vi "Gui_SetupExperiment.vi"(7 "Variant for Path":variant, 8 "error in (no error)":errorcluster, 11 "Variant":variant) -> (0 "error out":errorcluster caption="sortie d'erreur", 3 "Variant Output":variant)   [LabVIEW 2017]
uses:
  controls/LASER_Inputs.ctl
  controls/EXPERIMENT_Inputs.ctl
  controls/EXPERT_Path_Selector.ctl
panel:
  in  "EXPERIMENT Inputs":T1={"Setup"="", "Date"="", "User Name"="", "Comment"="", "Experiment Procedures"=[], "Chemical Source"="", "Sample Components"=[], "Species"=[], "Laser 1"={"Used"=FALSE, "Name"="", "Reference"="", "Wavelength"=0.0, "Energy"=0.0}, "Laser 2"={"Used"=FALSE, "Name"="", "Reference"="", "Wavelength"=0.0, "Energy"=0.0}, "Laser 3"={"Used"=FALSE, "Name"="", "Reference"="", "Wavelength"=0.0, "Energy"=0.0}, "Laser 4"={"Used"=TRUE, "Name"="Spectroscopy", "Reference"="Yag", "Wavelength"=1000.0, "Energy"=25.0}, "Laser 5"={"Used"=TRUE, "Name"="Spectroscopy", "Reference"="Yag", "Wavelength"=1000.0, "Energy"=25.0}, "Gas"=[]}
  in  "Gas":i32[](listbox)
  in  "Laser 5":T2={"Used"=TRUE, "Name"="Spectroscopy", "Reference"="Yag", "Wavelength"=1000.0, "Energy"=25.0}
  in  "Laser 4":T2={"Used"=TRUE, "Name"="Spectroscopy", "Reference"="Yag", "Wavelength"=1000.0, "Energy"=25.0}
  in  "Setup":string(combo)="PIRENEA"
  in  "Chemical Source":string(combo)="Christine JOBLIN"
  in  "Pre-Fill with default":bool
  out "Current Date":string
  in  "Laser 3":T2={"Used"=TRUE, "Name"="Spectroscopy", "Reference"="Yag", "Wavelength"=1000.0, "Energy"=25.0}
  in  "Laser 2":T2={"Used"=TRUE, "Name"="Spectroscopy", "Reference"="Yag", "Wavelength"=1000.0, "Energy"=25.0}
  in  "Laser 1":T2={"Used"=TRUE, "Name"="Spectroscopy", "Reference"="Yag", "Wavelength"=1000.0, "Energy"=25.0}
  in  "Comment":string
  in  "OK":bool
  in  "Species":i32[](listbox)
  in  "Sample Components":i32[](listbox)
  in  "Experiment Procedures":i32[](listbox)
  in  "User Name":string(combo)="Christine JOBLIN"
  # "Name"
  # "Reference"
  # "Wavelength"
  # "Energy"
  # "Name"
  # "Reference"
  # "(nm)"
  # "E (J)"
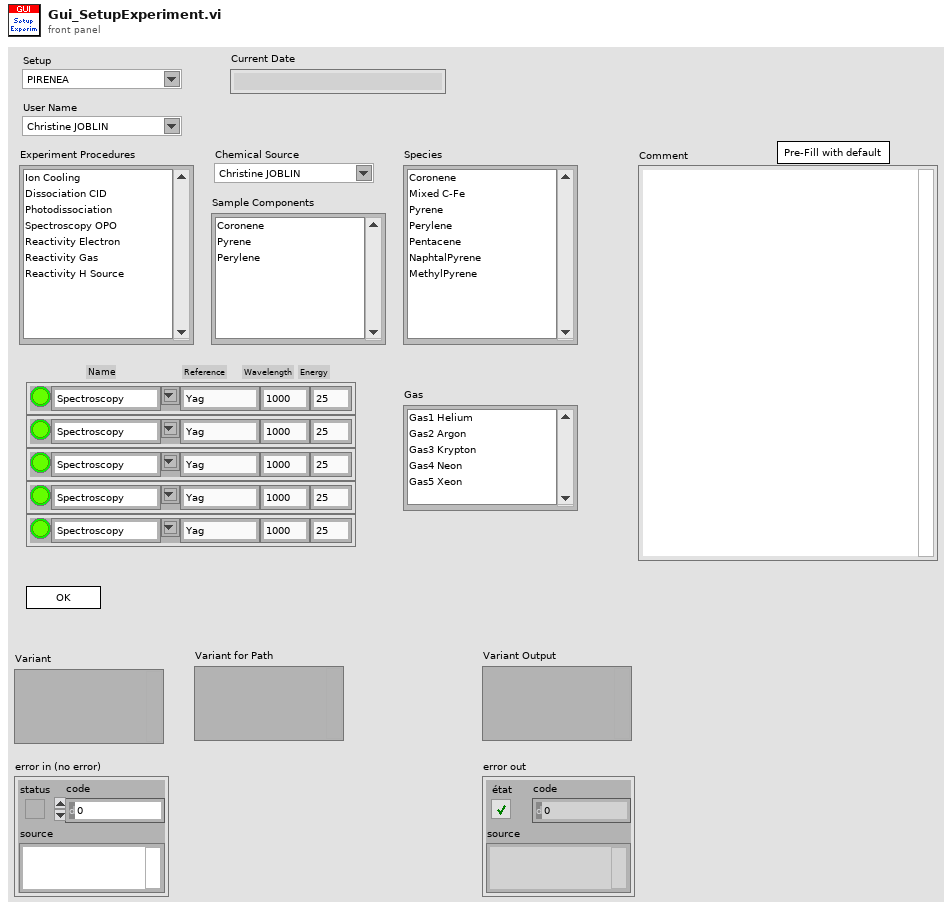
[diagram p1: front panel]
types:
  T1 = typedef "EXPERIMENT_Inputs.ctl" = cluster{"Setup":string, "Date":string, "User Name":string, "Comment":string, "Experiment Procedures":string[], "Chemical Source":string, "Sample Components":string[], "Species":string[], "Laser 1":T2, "Laser 2":T2, "Laser 3":T2, "Laser 4":T2, "Laser 5":T2, "Gas":string[]}
  T2 = typedef "LASER_Inputs.ctl" = cluster{"Used":bool, "Name":string, "Reference":string, "Wavelength":dbl, "Energy":dbl}
  T3 = typedef "EXPERT_Path_Selector.ctl" = enum16{"Application", "Resources", "Data", "XML", "XML Saved"}
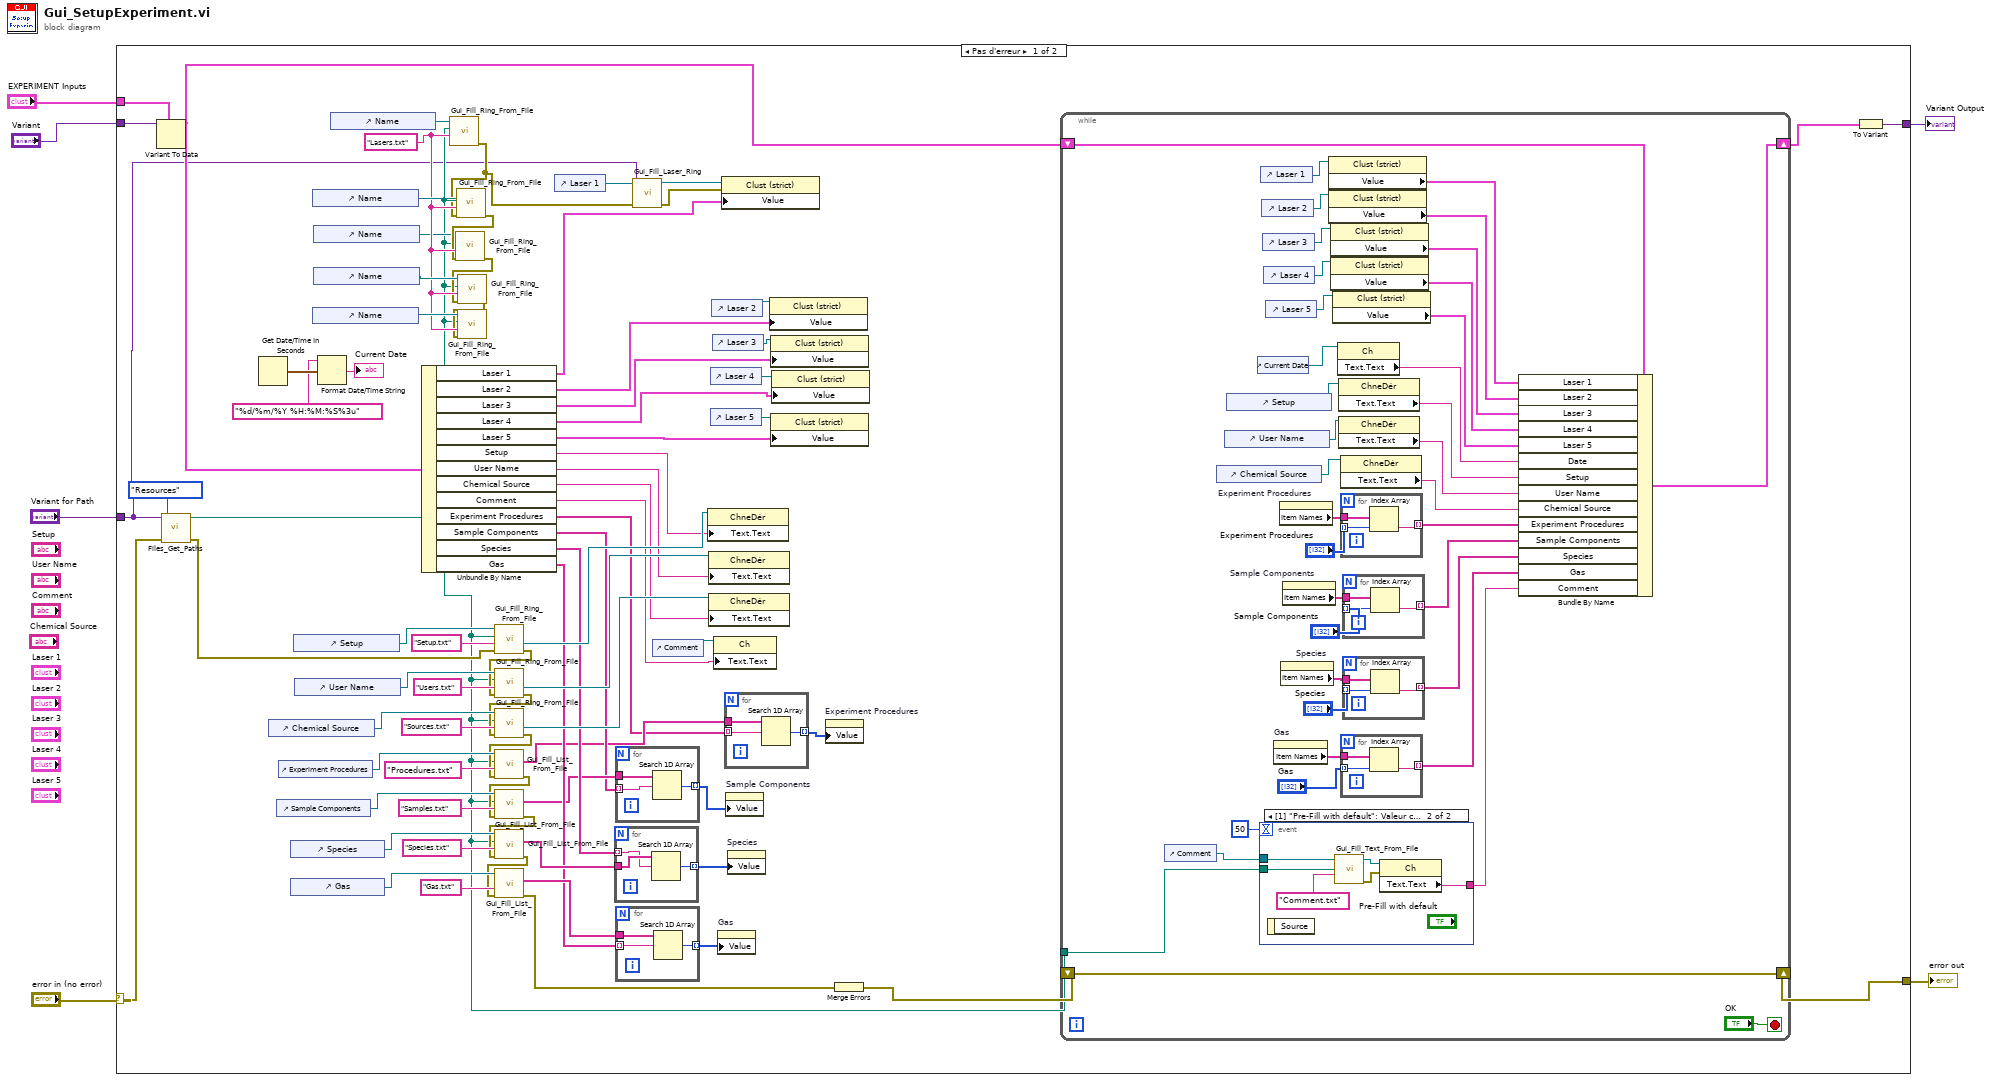
[diagram p0: block diagram]
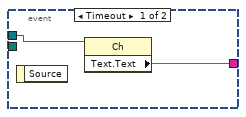
[diagram p2: hidden frame]
diagram:
  n1 = case shown="Pas d'erreur" "error in (no error)" {
    selector: "error in (no error)" -> [w43 w155]
    tunnel: [w69 w155] -> w6
    tunnel: "Variant" -> [w73 w156]
    tunnel: [w71 w156] -> w4
    tunnel: "Variant for Path" -> [w11 _]
    tunnel: "EXPERIMENT Inputs" -> [w29 _]
    frame No Error {
      w44 = "Lasers.txt" ("Resource Name")
      n2 = Variant To Data(type=w29, Variant=w73) -> (data=w72:T1)  [unwired: 1 in, 1 out]
      n3 = call "Files_Get_Paths.vi"("error in (no error)"=w43, "EXPERT Path Selector"=EXPERT_Path_Selector."Resources", "Variant"=w11) -> ("error out"=w41:errorcluster, "Path"=w13:path)  [unwired: 7 in]
      n4 = Get Date/Time In Seconds ("Date et heure en secondes")() -> (seconds since 1Jan1904=w76:timestamp)
      n5 = control-ref of="Chemical Source"() -> (w64:refnum<vi>)
      n6 = control-ref of="Sample Components"() -> (w82:refnum<vi>)
      n7 = control-ref of="Experiment Procedures"() -> (w83:refnum<vi>)
      n8 = control-ref of="Species"() -> (w81:refnum<vi>)
      n9 = control-ref of="Gas"() -> (w57:refnum<vi>)
      n10 = control-ref of="Setup"() -> (w66:refnum<vi>)
      n11 = control-ref of="User Name"() -> (w84:refnum<vi>)
      n12 = control-ref of="Name"() -> (w55:refnum<vi>)
      n13 = control-ref of="Name"() -> (w45:refnum<vi>)
      n14 = control-ref of="Name"() -> (w15:refnum<vi>)
      n15 = control-ref of="Name"() -> (w46:refnum<vi>)
      n16 = Format Date/Time String(time format string (%c)="%d/%m/%Y %H:%M:%S%3u" ("chaîne de format de l'heure (%c)"), seconds (now)=w76) -> (date/time string=→"Current Date":string)  [unwired: 1 in]
      n17 = control-ref of="Name"() -> (w7:refnum<vi>)
      n18 = Unbundle By Name(w72) -> ("Laser 1"=w9:T2, "Laser 2"=w51:T2, "Laser 3"=w50:T2, "Laser 4"=w49:T2, "Laser 5"=w25:T2, "Setup"=w62:string, "User Name"=w61:string, "Chemical Source"=w56:string, "Comment"=w59:string, "Experiment Procedures"=w17:string[], "Sample Components"=w20:string[], "Species"=w28:string[], "Gas"=w23:string[])
      n19 = call "Gui_Fill_Ring_From_File.vi"("Resource Name"=w44, "Resource Path"=w13, "Refnum ChneDér"=w7) -> ("error out"=w12:errorcluster)  [unwired: 5 in, 3 out]
      n20 = call "Gui_Fill_Ring_From_File.vi"("error in (no error)"=w12, "Resource Name"=w44, "Resource Path"=w13, "Refnum ChneDér"=w55) -> ("error out"=w33:errorcluster)  [unwired: 4 in, 3 out]
      n21 = call "Gui_Fill_Ring_From_File.vi"("error in (no error)"=w33, "Resource Name"=w44, "Resource Path"=w13, "Refnum ChneDér"=w15) -> ("error out"=w32:errorcluster)  [unwired: 4 in, 3 out]
      n22 = call "Gui_Fill_Ring_From_File.vi"("error in (no error)"=w32, "Resource Name"=w44, "Resource Path"=w13, "Refnum ChneDér"=w46) -> ("error out"=w31:errorcluster)  [unwired: 4 in, 3 out]
      n23 = call "Gui_Fill_Ring_From_File.vi"("error in (no error)"=w31, "Resource Name"=w44, "Resource Path"=w13, "Refnum ChneDér"=w45) -> ()  [unwired: 4 in, 4 out]
      n24 = call "Gui_Fill_Ring_From_File.vi"("error in (no error)"=w41, "Resource Name"="Setup.txt" ("nom ou chemin relatif"), "Resource Path"=w13, "Refnum ChneDér"=w66) -> ("error out"=w35:errorcluster, "Refnum ChneDér 2"=w63:refnum<vi>)  [unwired: 4 in, 2 out]
      n25 = call "Gui_Fill_Ring_From_File.vi"("error in (no error)"=w35, "Resource Name"="Users.txt" ("nom ou chemin relatif"), "Resource Path"=w13, "Refnum ChneDér"=w84) -> ("error out"=w36:errorcluster, "Refnum ChneDér 2"=w74:refnum<vi>)  [unwired: 4 in, 2 out]
      n26 = call "Gui_Fill_Ring_From_File.vi"("error in (no error)"=w36, "Resource Name"="Sources.txt" ("nom ou chemin relatif"), "Resource Path"=w13, "Refnum ChneDér"=w64) -> ("error out"=w37:errorcluster, "Refnum ChneDér 2"=w60:refnum<vi>)  [unwired: 4 in, 2 out]
      n27 = call "Gui_Fill_List_From_File.vi"("error in (no error)"=w37, "Resource Name"="Procedures.txt", "Resource Path"=w13, "Refnum LstDér"=w83) -> ("error out"=w38:errorcluster, "Table"=w18:string[])  [unwired: 5 in, 1 out]
      n28 = call "Gui_Fill_List_From_File.vi"("error in (no error)"=w38, "Resource Name"="Samples.txt", "Resource Path"=w13, "Refnum LstDér"=w82) -> ("error out"=w39:errorcluster, "Table"=w21:string[])  [unwired: 5 in, 1 out]
      n29 = call "Gui_Fill_List_From_File.vi"("error in (no error)"=w39, "Resource Name"="Species.txt", "Resource Path"=w13, "Refnum LstDér"=w81) -> ("error out"=w40:errorcluster, "Table"=w27:string[])  [unwired: 5 in, 1 out]
      n30 = call "Gui_Fill_List_From_File.vi"("error in (no error)"=w40, "Resource Name"="Gas.txt", "Refnum LstDér"=w57) -> ("error out"=w34:errorcluster, "Table"=w24:string[])  [unwired: 6 in, 1 out]
      n31 = control-ref of="Laser 1"() -> (w14:refnum<vi>)
      n32 = for {
        tunnel: w28 -> [w95] mode=indexing
        tunnel: w27 -> [w96]
        tunnel: [w94] -> w26 mode=indexing
        n33 = Search 1D Array(1D array=w96, element=w95) -> (index of element=w94:i32)  [unwired: 1 in]
      }
      n34 = for {
        tunnel: [w90] -> w19 mode=indexing
        tunnel: w21 -> [w89]
        tunnel: w20 -> [w88] mode=indexing
        n35 = Search 1D Array(1D array=w89, element=w88) -> (index of element=w90:i32)  [unwired: 1 in]
      }
      n36 = for {
        tunnel: [w93] -> w22 mode=indexing
        tunnel: w24 -> [w92]
        tunnel: w23 -> [w91] mode=indexing
        n37 = Search 1D Array(1D array=w92, element=w91) -> (index of element=w93:i32)  [unwired: 1 in]
      }
      n38 = call "Gui_Fill_Laser_Ring.vi"("Refnum Clust"=w14, "Variant for Path"=w11, "error in (no error)"=w12) -> ("Refnum Clust Out"=w10:refnum<vi>, "error out"=w8:errorcluster)  [unwired: 6 in]
      n39 = control-ref of="Comment"() -> (w68:refnum<vi>)
      n40 = property class="ChneDér"(reference=w63, "Text.Text"=w62) -> ()  [unwired: 1 in, 2 out]
      n41 = property class="ChneDér"(reference=w74, "Text.Text"=w61) -> ()  [unwired: 1 in, 2 out]
      n42 = property class="ChneDér"(reference=w60, "Text.Text"=w56) -> ()  [unwired: 1 in, 2 out]
      n43 = control-ref of="Laser 4"() -> (w47:refnum<vi>)
      n44 = control-ref of="Laser 5"() -> (w48:refnum<vi>)
      n45 = control-ref of="Laser 2"() -> (w53:refnum<vi>)
      n46 = control-ref of="Laser 3"() -> (w52:refnum<vi>)
      n47 = property class="Ch"(reference=w68, "Text.Text"=w59) -> ()  [unwired: 1 in, 2 out]
      n48 = property on="Gas" class="LstDér (strict)"("Value"=w22) -> ()  [unwired: 2 in, 2 out]
      n49 = property class="Clust (strict)"(reference=w10, error in=w8, "Value"=w9) -> ()  [unwired: 2 out]
      n50 = for {
        tunnel: [w87] -> w16 mode=indexing
        tunnel: w18 -> [w86]
        tunnel: w17 -> [w85] mode=indexing
        n51 = Search 1D Array(1D array=w86, element=w85) -> (index of element=w87:i32)  [unwired: 1 in]
      }
      n52 = property on="Sample Components" class="LstDér (strict)"("Value"=w19) -> ()  [unwired: 2 in, 2 out]
      n53 = property on="Species" class="LstDér (strict)"("Value"=w26) -> ()  [unwired: 2 in, 2 out]
      n54 = property class="Clust (strict)"(reference=w53, "Value"=w51) -> ()  [unwired: 1 in, 2 out]
      n55 = property class="Clust (strict)"(reference=w52, "Value"=w50) -> ()  [unwired: 1 in, 2 out]
      n56 = property class="Clust (strict)"(reference=w48, "Value"=w25) -> ()  [unwired: 1 in, 2 out]
      n57 = property class="Clust (strict)"(reference=w47, "Value"=w49) -> ()  [unwired: 1 in, 2 out]
      n58 = property on="Experiment Procedures" class="LstDér (strict)"("Value"=w16) -> ()  [unwired: 2 in, 2 out]
      n59 = Merge Errors(w34) -> (w70:errorcluster)
      n60 = while {
        shift-right: [w133] -> w54
        shift-left: w72 -> [w134]
        shift-right: [w122] -> w69
        shift-left: w70 -> [w122]
        tunnel: w13 -> [w121]
        stop <- "OK" stop-if-true
        n61 = control-ref of="Comment"() -> (w119:refnum<vi>)
        n62 = control-ref of="Chemical Source"() -> (w113:refnum<vi>)
        n63 = control-ref of="User Name"() -> (w114:refnum<vi>)
        n64 = control-ref of="Setup"() -> (w115:refnum<vi>)
        n65 = control-ref of="Current Date"() -> (w118:refnum<vi>)
        n66 = event shown="[1] \"Pre-Fill with default\": Valeur changée" {
          selector: _ -> [_ _]
          dyn-events: _ -> [_ _]
          timeout: 50 -> [_ _]
          tunnel: w121 -> [_ w142]
          tunnel: [w139 w141] -> w117
          tunnel: w119 -> [w138 w140]
          event Timeout {
            n67 = event-data() -> ()  [unwired: 1 in, 1 out]
            n68 = property class="Ch"(reference=w138) -> ("Text.Text"=w139:string)  [unwired: 1 in, 2 out]
          }
          event "Pre-Fill with default": Value Change {
            n69 = event-data() -> ()  [unwired: 1 in, 1 out]
            n70 = call "Gui_Fill_Text_From_File.vi"("Resource Name"="Comment.txt", "Resource Path"=w142, "Refnum Ch"=w140) -> ("error out"=w143:errorcluster, "Refnum Ch out"=w144:refnum<vi>)  [unwired: 7 in]
            n71 = property class="Ch"(reference=w144, error in=w143) -> ("Text.Text"=w141:string)  [unwired: 2 out]
          }
        }
        n72 = control-ref of="Laser 1"() -> (w109:refnum<vi>)
        n73 = control-ref of="Laser 2"() -> (w108:refnum<vi>)
        n74 = control-ref of="Laser 3"() -> (w107:refnum<vi>)
        n75 = control-ref of="Laser 4"() -> (w106:refnum<vi>)
        n76 = control-ref of="Laser 5"() -> (w105:refnum<vi>)
        n77 = property on="Gas" class="LstDér (strict)"() -> ("Item Names"=w99:string[])  [unwired: 2 in, 2 out]
        n78 = property on="Experiment Procedures" class="LstDér (strict)"() -> ("Item Names"=w131:string[])  [unwired: 2 in, 2 out]
        n79 = property on="Species" class="LstDér (strict)"() -> ("Item Names"=w126:string[])  [unwired: 2 in, 2 out]
        n80 = property on="Sample Components" class="LstDér (strict)"() -> ("Item Names"=w128:string[])  [unwired: 2 in, 2 out]
        n81 = property class="Clust (strict)"(reference=w109) -> ("Value"=w100:T2)  [unwired: 1 in, 2 out]
        n82 = property class="Clust (strict)"(reference=w108) -> ("Value"=w101:T2)  [unwired: 1 in, 2 out]
        n83 = property class="Clust (strict)"(reference=w107) -> ("Value"=w102:T2)  [unwired: 1 in, 2 out]
        n84 = property class="Clust (strict)"(reference=w106) -> ("Value"=w103:T2)  [unwired: 1 in, 2 out]
        n85 = property class="Clust (strict)"(reference=w105) -> ("Value"=w104:T2)  [unwired: 1 in, 2 out]
        n86 = property class="Ch"(reference=w118) -> ("Text.Text"=w116:string)  [unwired: 1 in, 2 out]
        n87 = property class="ChneDér"(reference=w115) -> ("Text.Text"=w111:string)  [unwired: 1 in, 2 out]
        n88 = property class="ChneDér"(reference=w114) -> ("Text.Text"=w110:string)  [unwired: 1 in, 2 out]
        n89 = property class="ChneDér"(reference=w113) -> ("Text.Text"=w112:string)  [unwired: 1 in, 2 out]
        n90 = for {
          tunnel: [w154] -> w129 mode=indexing
          tunnel: w131 -> [w153]
          tunnel: "Experiment Procedures" -> [w152] mode=indexing
          n91 = Index Array(array=w153, index=w152) -> (element=w154:string)
        }
        n92 = for {
          tunnel: [w137] -> w98 mode=indexing
          tunnel: "Gas" -> [w136] mode=indexing
          tunnel: w99 -> [w135]
          n93 = Index Array(array=w135, index=w136) -> (element=w137:string)
        }
        n94 = for {
          tunnel: [w151] -> w124 mode=indexing
          tunnel: w128 -> [w150]
          tunnel: "Sample Components" -> [w149] mode=indexing
          n95 = Index Array(array=w150, index=w149) -> (element=w151:string)
        }
        n96 = for {
          tunnel: [w148] -> w123 mode=indexing
          tunnel: w126 -> [w147]
          tunnel: "Species" -> [w146] mode=indexing
          n97 = Index Array(array=w147, index=w146) -> (element=w148:string)
        }
        n98 = Bundle By Name(cluster=w134, "Laser 1"=w100, "Laser 2"=w101, "Laser 3"=w102, "Laser 4"=w103, "Laser 5"=w104, "Date"=w116, "Setup"=w111, "User Name"=w110, "Chemical Source"=w112, "Experiment Procedures"=w129, "Sample Components"=w124, "Species"=w123, "Gas"=w98, "Comment"=w117) -> (w133:T1)
      }
      n99 = To Variant(anything=w54) -> (Variant=w71:variant)
    }
    frame Error {
    }
  }
  "error out" <- w6
  "Variant Output" <- w4
